vi "SSC DCPower Configure Output Enabled And Connected.vi"(0 "DCPower SSC in":T1[](array[typedef]), 5 "Output Enabled And Connected":bool, 11 "error in":errorcluster, 12 "Delay Before/After VDD":dbl format="%#_6p") -> (4 "DCPower SSC out":T1[](array[typedef]), 15 "error out":errorcluster)   [LabVIEW 2019]
doc: "This VI configures output enabled and connected on the channels.\n\nT - Enable and then connect\nF - Disconnect and then disable"
uses:
  SSC DCPower.ctl
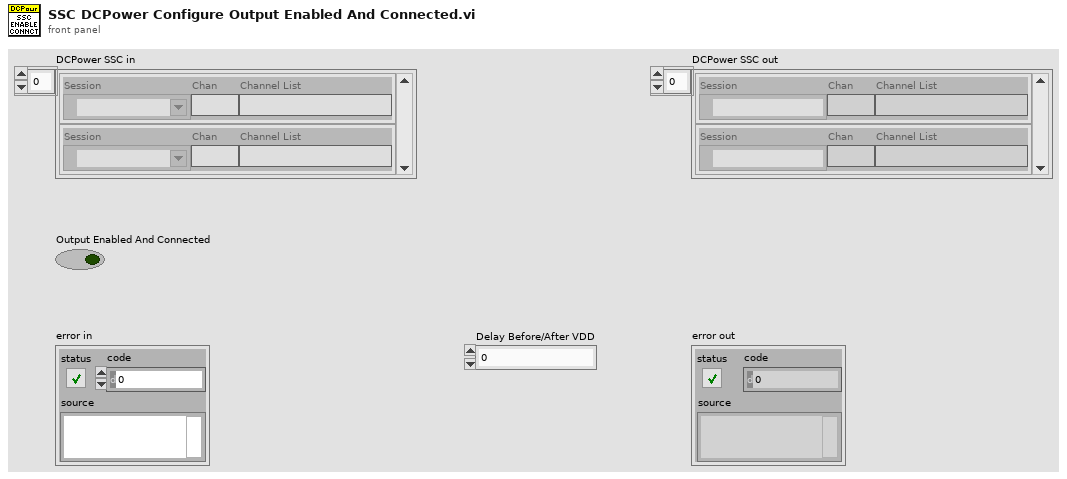
[diagram p1: front panel]
types:
  T1 = typedef "SSC DCPower.ctl" = cluster{"Session":refnum<k15>, "Chan":string, "Channel List":string}
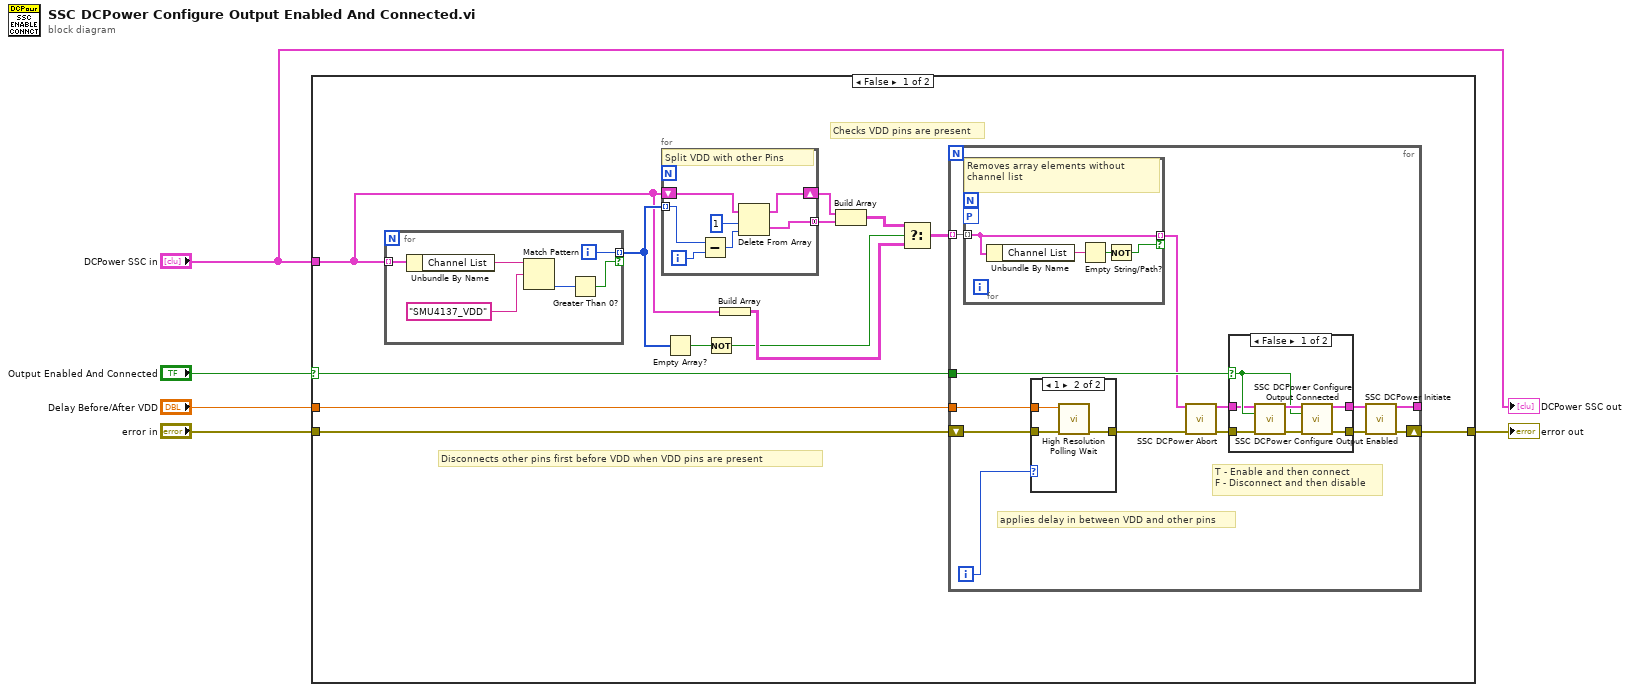
[diagram p0: block diagram]
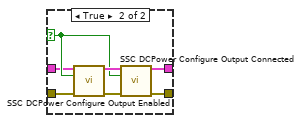
[diagram p3: hidden frame]
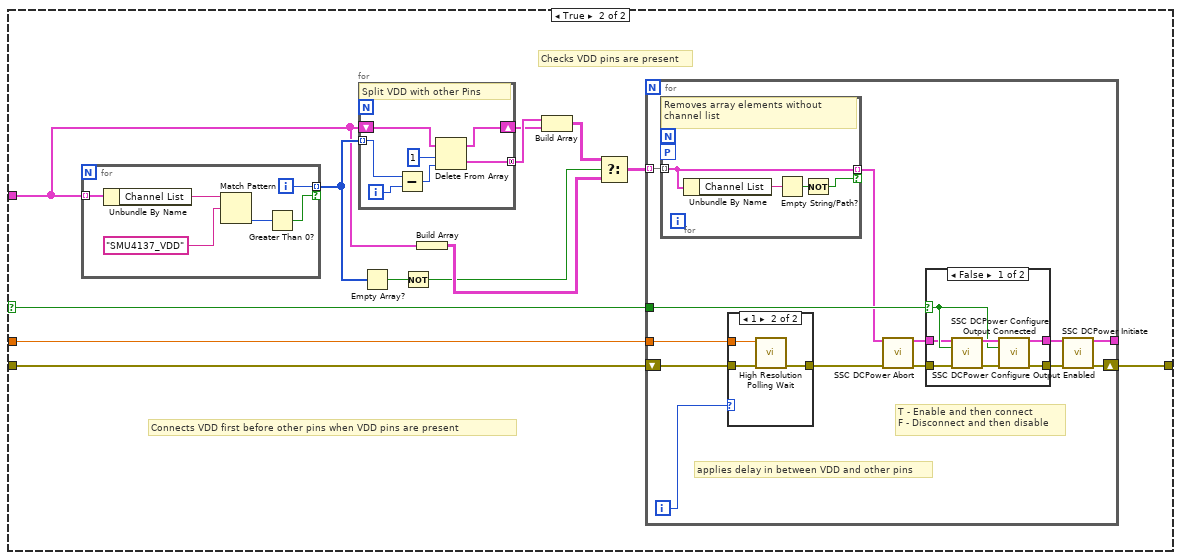
[diagram p4: hidden frame]
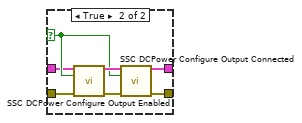
[diagram p6: hidden frame]
diagram:
  n1 = case shown="False" "Output Enabled And Connected" {
    selector: "Output Enabled And Connected" -> [w7 w70]
    tunnel: "error in" -> [w12 w73]
    tunnel: [w10 w71] -> w4
    tunnel: "DCPower SSC in" -> [w11 w72]
    tunnel: "Delay Before/After VDD" -> [w6 w69]
    frame False {
      # "Disconnects other pins first before VDD when VDD pins are present"
      # "Checks VDD pins are present"
      n2 = for {
        tunnel: w11 -> [w31] mode=indexing
        tunnel: [w27] -> w18 mode=indexing if=w26
        i -> [w27]
        n3 = Unbundle By Name(w31) -> ("Channel List"=w30:string)
        n4 = Match Pattern(string=w30, regular expression="SMU4137_VDD") -> (offset past match=w28:i32)  [unwired: 1 in, 3 out]
        n5 = Greater Than 0?(x=w28) -> (x > 0?=w26:bool)
      }
      n6 = for {
        shift-right: [w22] -> w9
        shift-left: w11 -> [w25]
        tunnel: w18 -> [w21] mode=indexing
        tunnel: [w24] -> w8 mode=concatenating
        i -> [w19]
        # "Split VDD with other Pins"
        n7 = Subtract(x=w21, y=w19) -> (x-y=w20:i32)
        n8 = Delete From Array(array=w25, length=1, index=w20) -> (deleted portion=w24:T1[], array with subset deleted=w22:T1[])
      }
      n9 = Empty Array?(array=w18) -> (empty?=w17:bool)
      n10 = Not(x=w17) -> (.not. x?=w14:bool)
      n11 = Build Array(w11) -> (w15:T1[][])
      n12 = Build Array(w9, w8) -> (w16:T1[][])
      n13 = Select(t=w16, s=w14, f=w15) -> (s? t:f=w13:T1[][])
      n14 = for {
        tunnel: [w35] -> _
        tunnel: w7 -> [w44]
        shift-right: [w37] -> w10
        shift-left: w12 -> [w42]
        tunnel: w13 -> [w43] mode=indexing
        tunnel: w6 -> [w33]
        i -> [w32]
        # "applies delay in between VDD and other pins"
        # "T - Enable and then connect\nF - Disconnect and then disable"
        n15 = for {
          tunnel: w43 -> [w52] mode=indexing
          workers-P: _ -> [_]
          tunnel: [w52] -> w40 mode=indexing if=w49
          # "Removes array elements without channel list"
          n16 = Unbundle By Name(w52) -> ("Channel List"=w50:string)
          n17 = Empty String/Path?(string/path=w50) -> (empty?=w51:bool)
          n18 = Not(x=w51) -> (.not. x?=w49:bool)
        }
        n19 = case shown="1" w32 {
          tunnel: w42 -> [w45 w48]
          tunnel: [w45 w47] -> w34
          tunnel: w33 -> [_ w46]
          frame 0, Default {
          }
          frame 1 {
            n20 = call <vilib>:"High Resolution Polling Wait.vi"("error in (no error)"=w48, "seconds to wait"=w46) -> ("error out"=w47:errorcluster)  [unwired: 9 in]
          }
        }
        n21 = call "SSC DCPower Abort.vi"("DCPower SSC in"=w40, "error in"=w34) -> ("DCPower SSC out"=w39:T1[], "error out"=w41:errorcluster)  [unwired: 12 in]
        n22 = case shown="False" w44 {
          selector: w44 -> [w54 w61]
          tunnel: w41 -> [w59 w66]
          tunnel: [w57 w64] -> w38
          tunnel: [w55 w62] -> w36
          tunnel: w39 -> [w53 w60]
          frame False {
            n23 = call "SSC DCPower Configure Output Connected.vi"("DCPower SSC in"=w53, "Output Connected"=w54, "error in"=w59) -> ("DCPower SSC out"=w56:T1[], "error out"=w58:errorcluster)  [unwired: 11 in]
            n24 = call "SSC DCPower Configure Output Enabled.vi"("DCPower SSC in"=w56, "Output Enabled"=w54, "error in"=w58) -> ("DCPower SSC out"=w55:T1[], "error out"=w57:errorcluster)  [unwired: 11 in]
          }
          frame True {
            n25 = call "SSC DCPower Configure Output Enabled.vi"("DCPower SSC in"=w60, "Output Enabled"=w61, "error in"=w66) -> ("DCPower SSC out"=w63:T1[], "error out"=w65:errorcluster)  [unwired: 11 in]
            n26 = call "SSC DCPower Configure Output Connected.vi"("DCPower SSC in"=w63, "Output Connected"=w61, "error in"=w65) -> ("DCPower SSC out"=w62:T1[], "error out"=w64:errorcluster)  [unwired: 11 in]
          }
        }
        n27 = call "SSC DCPower Initiate.vi"("DCPower SSC in"=w36, "error in"=w38) -> ("DCPower SSC out"=w35:T1[], "error out"=w37:errorcluster)  [unwired: 12 in]
      }
    }
    frame True {
      # "Connects VDD first before other pins when VDD pins are present"
      # "Checks VDD pins are present"
      n28 = for {
        tunnel: w72 -> [w92] mode=indexing
        tunnel: [w88] -> w79 mode=indexing if=w87
        i -> [w88]
        n29 = Unbundle By Name(w92) -> ("Channel List"=w91:string)
        n30 = Match Pattern(string=w91, regular expression="SMU4137_VDD") -> (offset past match=w89:i32)  [unwired: 1 in, 3 out]
        n31 = Greater Than 0?(x=w89) -> (x > 0?=w87:bool)
      }
      n32 = for {
        shift-right: [w83] -> w67
        shift-left: w72 -> [w86]
        tunnel: w79 -> [w82] mode=indexing
        tunnel: [w85] -> w68 mode=concatenating
        i -> [w80]
        # "Split VDD with other Pins"
        n33 = Subtract(x=w82, y=w80) -> (x-y=w81:i32)
        n34 = Delete From Array(array=w86, length=1, index=w81) -> (deleted portion=w85:T1[], array with subset deleted=w83:T1[])
      }
      n35 = Empty Array?(array=w79) -> (empty?=w78:bool)
      n36 = Not(x=w78) -> (.not. x?=w75:bool)
      n37 = Build Array(w72) -> (w76:T1[][])
      n38 = Build Array(w68, w67) -> (w77:T1[][])
      n39 = Select(t=w77, s=w75, f=w76) -> (s? t:f=w74:T1[][])
      n40 = for {
        tunnel: [w96] -> _
        tunnel: w70 -> [w105]
        shift-right: [w98] -> w71
        shift-left: w73 -> [w103]
        tunnel: w74 -> [w104] mode=indexing
        tunnel: w69 -> [w94]
        i -> [w93]
        # "applies delay in between VDD and other pins"
        # "T - Enable and then connect\nF - Disconnect and then disable"
        n41 = for {
          tunnel: w104 -> [w113] mode=indexing
          workers-P: _ -> [_]
          tunnel: [w113] -> w101 mode=indexing if=w110
          # "Removes array elements without channel list"
          n42 = Unbundle By Name(w113) -> ("Channel List"=w111:string)
          n43 = Empty String/Path?(string/path=w111) -> (empty?=w112:bool)
          n44 = Not(x=w112) -> (.not. x?=w110:bool)
        }
        n45 = case shown="1" w93 {
          tunnel: w103 -> [w106 w109]
          tunnel: [w106 w108] -> w95
          tunnel: w94 -> [_ w107]
          frame 0, Default {
          }
          frame 1 {
            n46 = call <vilib>:"High Resolution Polling Wait.vi"("error in (no error)"=w109, "seconds to wait"=w107) -> ("error out"=w108:errorcluster)  [unwired: 9 in]
          }
        }
        n47 = call "SSC DCPower Abort.vi"("DCPower SSC in"=w101, "error in"=w95) -> ("DCPower SSC out"=w100:T1[], "error out"=w102:errorcluster)  [unwired: 12 in]
        n48 = case shown="False" w105 {
          selector: w105 -> [w115 w122]
          tunnel: w102 -> [w120 w127]
          tunnel: [w118 w125] -> w99
          tunnel: [w116 w123] -> w97
          tunnel: w100 -> [w114 w121]
          frame False {
            n49 = call "SSC DCPower Configure Output Connected.vi"("DCPower SSC in"=w114, "Output Connected"=w115, "error in"=w120) -> ("DCPower SSC out"=w117:T1[], "error out"=w119:errorcluster)  [unwired: 11 in]
            n50 = call "SSC DCPower Configure Output Enabled.vi"("DCPower SSC in"=w117, "Output Enabled"=w115, "error in"=w119) -> ("DCPower SSC out"=w116:T1[], "error out"=w118:errorcluster)  [unwired: 11 in]
          }
          frame True {
            n51 = call "SSC DCPower Configure Output Enabled.vi"("DCPower SSC in"=w121, "Output Enabled"=w122, "error in"=w127) -> ("DCPower SSC out"=w124:T1[], "error out"=w126:errorcluster)  [unwired: 11 in]
            n52 = call "SSC DCPower Configure Output Connected.vi"("DCPower SSC in"=w124, "Output Connected"=w122, "error in"=w126) -> ("DCPower SSC out"=w123:T1[], "error out"=w125:errorcluster)  [unwired: 11 in]
          }
        }
        n53 = call "SSC DCPower Initiate.vi"("DCPower SSC in"=w97, "error in"=w99) -> ("DCPower SSC out"=w96:T1[], "error out"=w98:errorcluster)  [unwired: 12 in]
      }
    }
  }
  "error out" <- w4
  "DCPower SSC out" <- "DCPower SSC in"
